vi "Initialize.vi"(0 "Display State In":T1, 9 "Container State":T2, 11 "error in (no error)":errorcluster) -> (4 "Display State Out":T1, 15 "error out":errorcluster)   [LabVIEW 2020, in "TTL XCtrl.xctl"]
uses:
  TTL XCtrl.xctl
  <vilib>/_xctls/Container State.ctl
  State.vi
  TTL VIs/Device Classes/Base Class/TTLControlledDevice.lvclass
  <vilib>/_xctls/XControlSupport.lvlib
types:
  T1 = typedef "TTL XCtrl.xctl/State.vi" = cluster{"Devices":refnum<class "TTLControlledDevice.lvclass">[], "action":string}
  T2 = typedef "XControlSupport.lvlib/Container State.ctl" = cluster{"Indicator?":bool, "Run Mode?":bool, " Refnum":refnum<vi>}
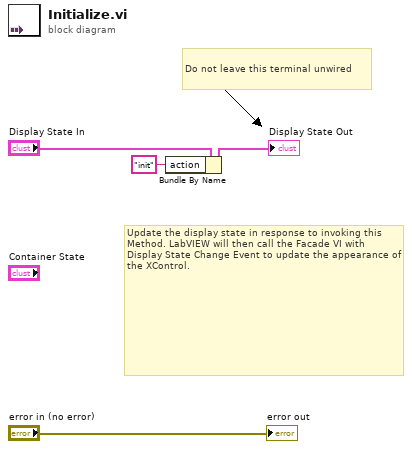
[diagram p0: block diagram]
diagram:
  # "Do not leave this terminal unwired"
  # "Update the display state in response to invoking this Method. LabVIEW will then call the Facade VI with Display State Change Event to update the appearance of the XControl."
  n1 = Bundle By Name(cluster="Display State In", "action"="init") -> (→"Display State Out":T1)
  "error out" <- "error in (no error)"
